vi "Read name.vi"(11 "TestManagerMsg.Measurement in":refnum<class "TestManagerMsg.Measurement.lvclass">) -> (2 "name":string, 3 "TestManagerMsg.Measurement out":refnum<class "TestManagerMsg.Measurement.lvclass">)   [LabVIEW 2013, in "Caraya.lvlib" / "TestManagerMsg.Measurement.lvclass"]
uses:
  TestManagerMsg.Measurement.lvclass
  TestManagerMsg.Measurement.lvclass/TestManagerMsg.Measurement.ctl
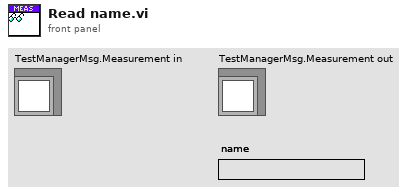
[diagram p1: front panel]
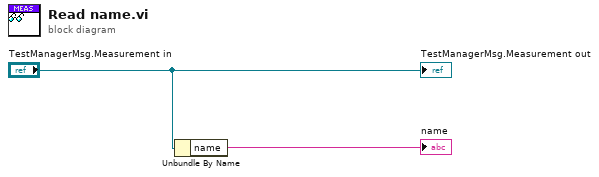
[diagram p0: block diagram]
diagram:
  n1 = Unbundle By Name("TestManagerMsg.Measurement in") -> ("name"=→"name":string)
  "TestManagerMsg.Measurement out" <- "TestManagerMsg.Measurement in"
